vi "Read VI Refnum.vi"(8 "error in (no error)":errorcluster, 11 "VI File in":refnum<class "VI File.lvclass">) -> (0 "error out":errorcluster, 2 "VI Refnum":refnum<vi>, 3 "VI File out":refnum<class "VI File.lvclass">)   [LabVIEW 2020, in "Save for Previous Version.lvlib" / "VI File.lvclass"]
uses:
  VI File.lvclass
  VI File.lvclass/VI File.ctl
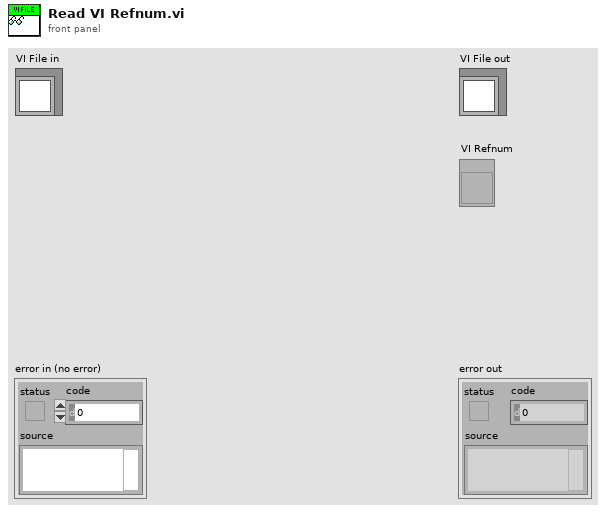
[diagram p1: front panel]
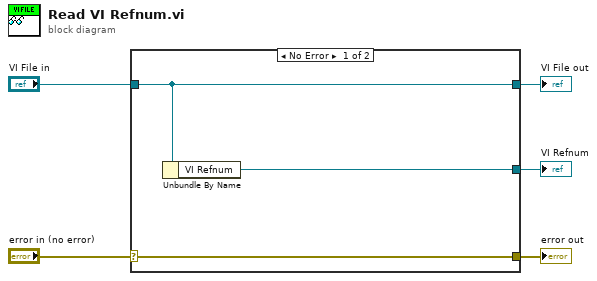
[diagram p0: block diagram]
diagram:
  n1 = case shown="No Error" "error in (no error)" {
    selector: "error in (no error)" -> [w8 w9]
    tunnel: [w8 w9] -> w4
    tunnel: [w7 w10] -> w2
    tunnel: "VI File in" -> [w7 w10]
    tunnel: [w6 _] -> w1
    frame No Error {
      n2 = Unbundle By Name(w7) -> ("VI Refnum"=w6:refnum<vi>)
    }
    frame Error {
    }
  }
  "error out" <- w4
  "VI File out" <- w2
  "VI Refnum" <- w1
